vi "Get Server Version.vi"(0 "InfluxDB in":refnum<class "Client.lvclass">, 11 "error in (no error)":errorcluster) -> (4 "InfluxDB out":refnum<class "Client.lvclass">, 6 "Version":string, 15 "error out":errorcluster)   [LabVIEW 2018, in "InfluxDB Client.lvlib" / "Client.lvclass"]
doc: "Creates a database."
uses:
  Client.lvclass
  Client.lvclass/Client.ctl
  <vilib>/httpClient/LabVIEWHTTPClient.lvlib
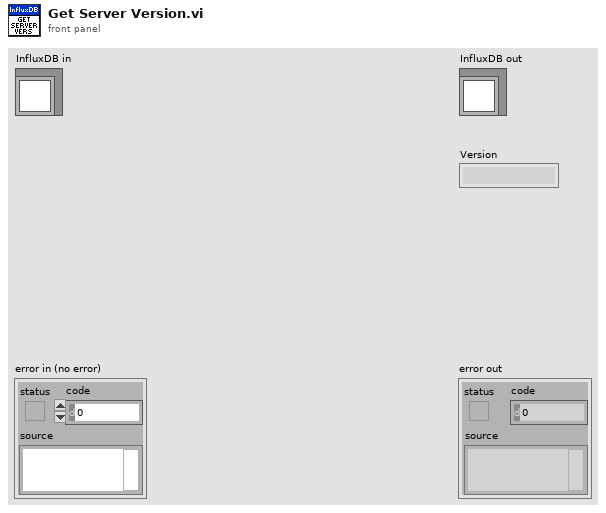
[diagram p1: front panel]
types:
  T1 = typedef "Dictionary Object RefNum__ogtk.ctl" = refnum<k1>
  T2 = typedef "LabVIEWHTTPClient.lvlib/ClientHandle.ctl" = refnum<k1>
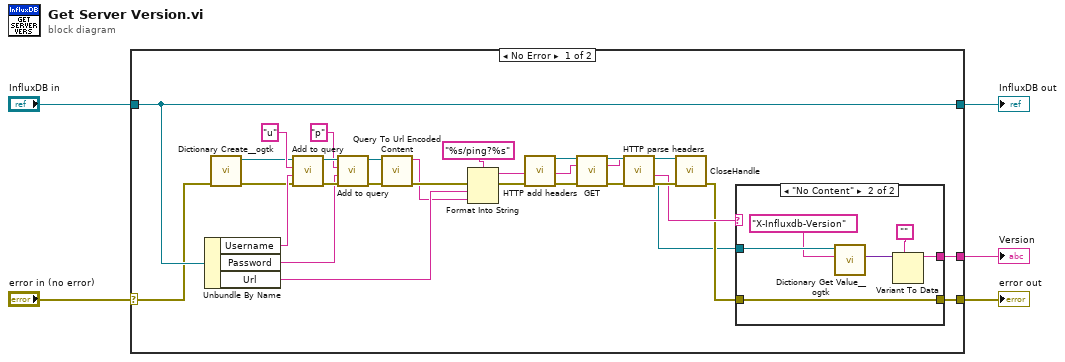
[diagram p0: block diagram]
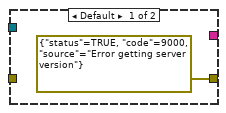
[diagram p2: hidden frame]
diagram:
  n1 = case shown="No Error" "error in (no error)" {
    selector: "error in (no error)" -> [w14 w42]
    tunnel: [w11 w42] -> w4
    tunnel: [w15 w41] -> w2
    tunnel: "InfluxDB in" -> [w15 w41]
    tunnel: [w6 _] -> w1
    frame No Error {
      n2 = Unbundle By Name(w15) -> ("Username"=w22:string, "Password"=w24:string, "Url"=w29:string)
      n3 = call <userlib>:"Dictionary Create__ogtk.vi"("error in (no error)"=w14) -> ("error out"=w17:errorcluster, "dictionary out"=w16:T1)  [unwired: 9 in]
      n4 = call "Add to query.vi"("error in (no error)"=w17, "Value"=w22, "Parameter"="u", "Query in"=w16) -> ("error out"=w31:errorcluster, "Query out"=w23:T1)  [unwired: 6 in]
      n5 = call "Add to query.vi"("error in (no error)"=w31, "Value"=w24, "Parameter"="p", "Query in"=w23) -> ("error out"=w32:errorcluster, "Query out"=w30:T1)  [unwired: 6 in]
      n6 = call "Query To Url Encoded Content.vi"("error in (no error)"=w32, "Query"=w30) -> ("error out"=w33:errorcluster, "Url Encoded Content"=w18:string)  [unwired: 8 in]
      n7 = Format Into String(format string="%s/ping?%s", error in=w33, w29, w18) -> (resulting string=w27:string, error out=w28:errorcluster)  [unwired: 1 in]
      n8 = call "HTTP add headers.vi"("error in (no error)"=w28) -> ("client handle out"=w10:T2, "error out"=w26:errorcluster)  [unwired: 13 in]
      n9 = call <vilib>:"GET.vi"("client handle"=w10, "url"=w27, "error in (no error)"=w26) -> ("client handle out"=w9:T2, "headers"=w7:string, "error out"=w25:errorcluster)  [unwired: 9 in, 1 out]
      n10 = call "HTTP parse headers.vi"("HTTP headers"=w7) -> ("Headers out"=w8:T1, "Status"=w13:string)  [unwired: 7 in, 2 out]
      n11 = call <vilib>:"CloseHandle.vi"("client handle"=w9, "error in (no error)"=w25) -> ("error out"=w12:errorcluster)  [unwired: 13 in]
      n12 = case shown="\"No Content\"" w13 {
        tunnel: w12 -> [_ w40]
        tunnel: [errorcluster {"status"=TRUE, "code"=9000, "source"="Error getting server version"} ("error out") w40] -> w11
        tunnel: w8 -> [_ w39]
        tunnel: [_ w35] -> w6
        frame Default {
        }
        frame "No Content" {
          n13 = call <userlib>:"Dictionary Get Value__ogtk.vi"("key"="X-Influxdb-Version", "dictionary"=w39) -> ("value"=w37:variant)  [unwired: 6 in, 3 out]
          n14 = Variant To Data(type="", Variant=w37) -> (data=w35:string)  [unwired: 1 in, 1 out]
        }
      }
    }
    frame Error {
    }
  }
  "error out" <- w4
  "InfluxDB out" <- w2
  "Version" <- w1
